vi "运维调试.vi"() -> ()   [LabVIEW 2016, in "重金属.lvlib"]
uses:
  <vilib>/Plasmionique/MB Master/MB_Master/MB_Master.lvclass
  <vilib>/Utility/miscctls.llb/LVPointTypeDef.ctl
  <userlib>/_OpenG.lib/array/array.llb/Remove Duplicates from 1D Array (String)__ogtk.vi
  <vilib>/Utility/config.llb/NI_LVConfig.lvlib
panel:
  out "MB session out":refnum<class "MB_Master.lvclass">
  out "测量结果":T1 {"汞" format="%.5f"; "锰" format="%.5f"; "镍" format="%.5f"; "锌" format="%.5f"; "铜" format="%.5f"; "镉" format="%.5f"; "铅" format="%.5f"}
  in  "参数选择配置":T2 {"通道4" items=["不启用", "铅", "镉", "铜", "锌", "镍", "锰", "汞"]; "通道3" items=["不启用", "铅", "镉", "铜", "锌", "镍", "锰", "汞"]; "通道2" items=["不启用", "铅", "镉", "铜", "锌", "镍", "锰", "汞"]; "通道1" items=["不启用", "铅", "镉", "铜", "锌", "镍", "锰", "汞"]}
  out "字符串":string
  in  "测试时间设置":dbl
  out "通讯状态":bool
  in  "设置":bool
  in  "停止":bool
  in  "启动":bool
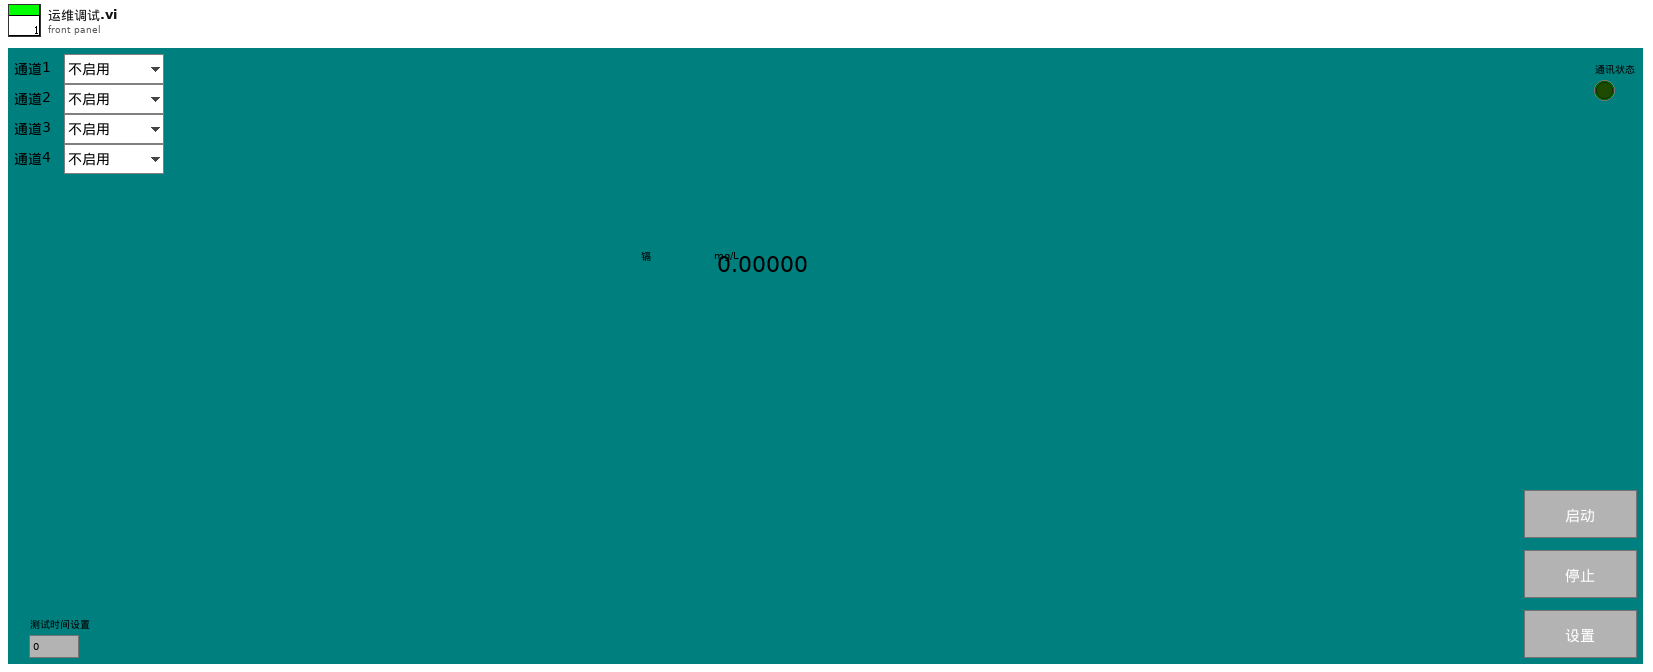
[diagram p1: front panel]
types:
  T1 = cluster{"铅":sgl, "镉":sgl, "铜":sgl, "锌":sgl, "镍":sgl, "锰":sgl, "汞":sgl}
  T2 = cluster{"通道1":u16, "通道2":u16, "通道3":u16, "通道4":u16}
  T3 = typedef "LVPointTypeDef.ctl" = cluster{"Horizontal":i16, "Vertical":i16}
  T4 = typedef "NI_LVConfig.lvlib/Config Data RefNum.ctl" = refnum<k1>
  T5 = cluster{"连接类型":enum16{"串口", "TCP"}, "串口":string, "IP":string, "PORT":string}
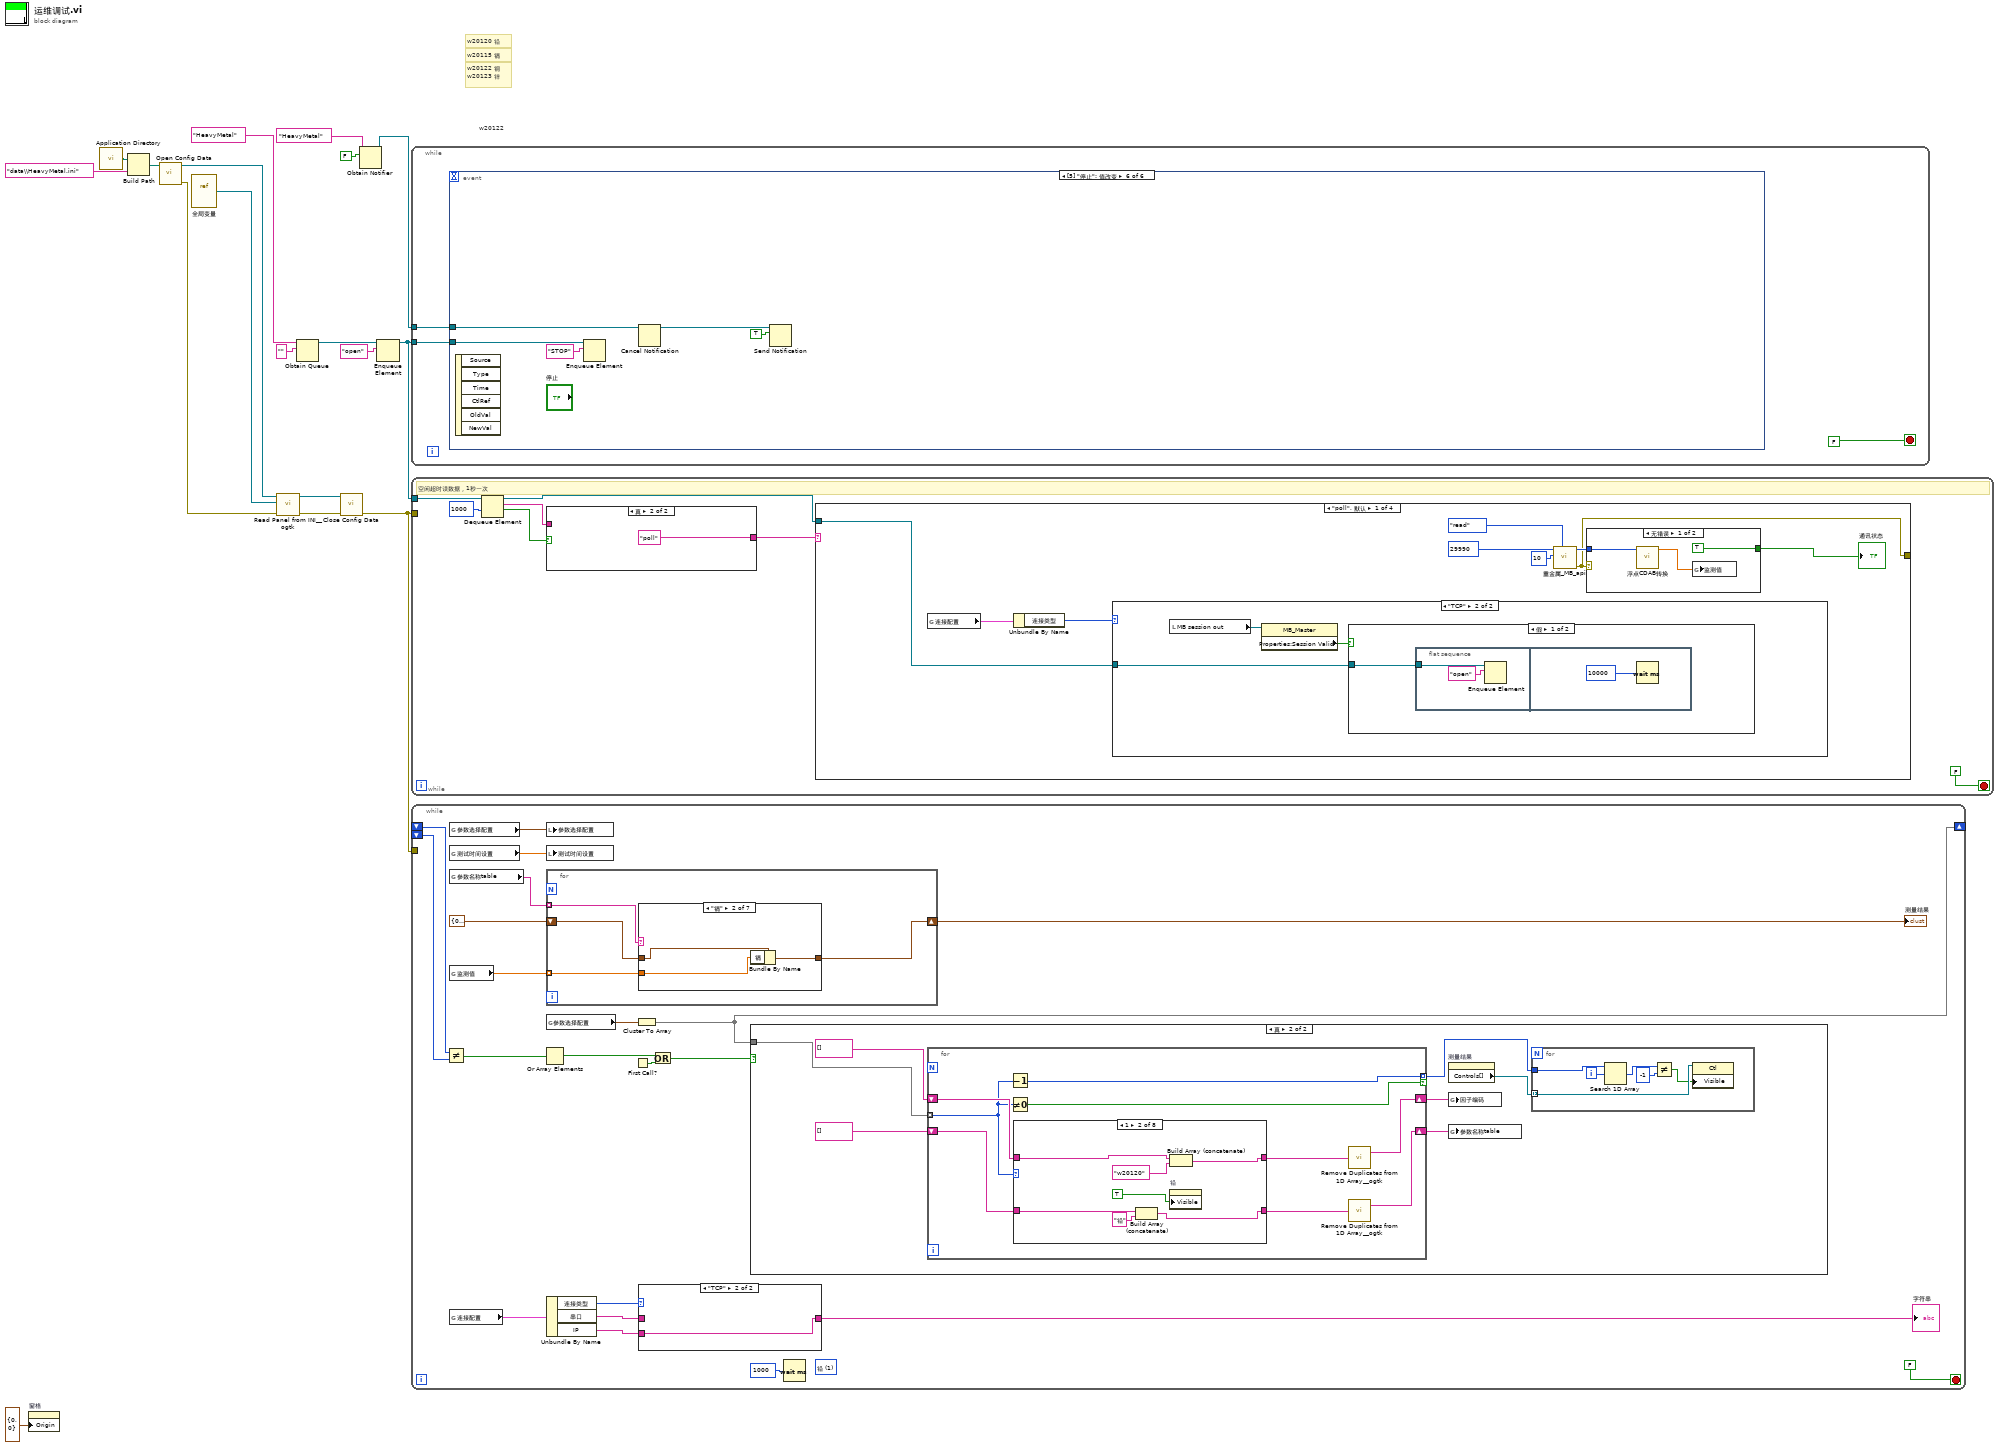
[diagram p0: block diagram]
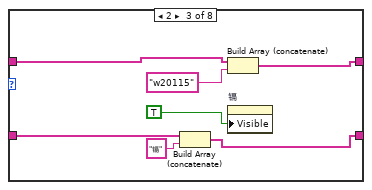
[diagram p4: hidden frame]
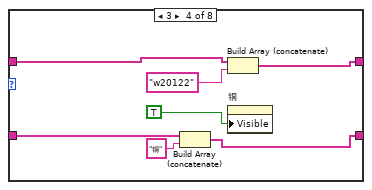
[diagram p5: hidden frame]
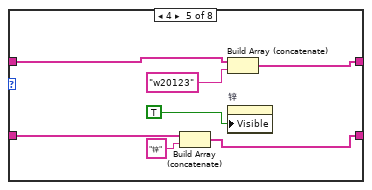
[diagram p6: hidden frame]
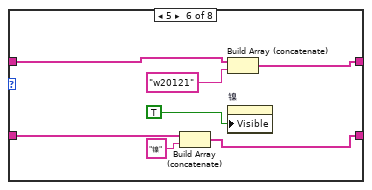
[diagram p7: hidden frame]
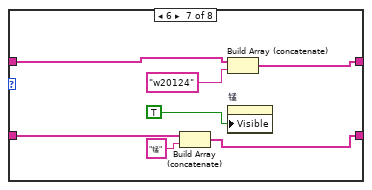
[diagram p8: hidden frame]
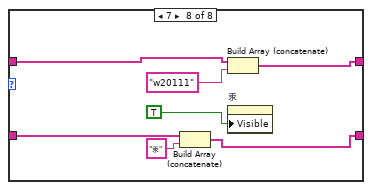
[diagram p9: hidden frame]
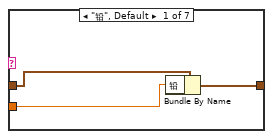
[diagram p11: hidden frame]
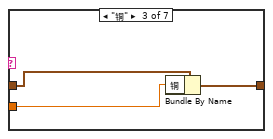
[diagram p12: hidden frame]
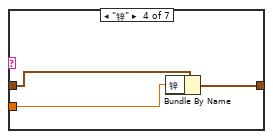
[diagram p13: hidden frame]
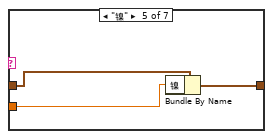
[diagram p14: hidden frame]
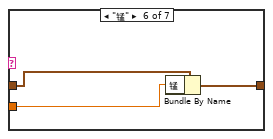
[diagram p15: hidden frame]
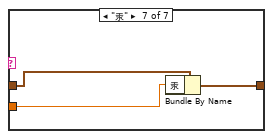
[diagram p16: hidden frame]
diagram:
  # "w20115\t镉"
  # "w20120\t铅"
  # "w20122\t铜\nw20123\t锌"
  # "w20122"
  n1 = property on="窗格" class="Pane"("Origin"=T3 {"Horizontal"=0, "Vertical"=0} ("原点")) -> ()  [unwired: 2 in, 2 out]
  n2 = call <vilib>:"Application Directory.vi"() -> ("Application Directory"=w6:path)
  n3 = Build Path(base path=w6, name or relative path="data\\HeavyMetal.ini" ("名称或相对路径")) -> (appended path=w8:path)
  n4 = call <vilib>:"Open Config Data.vi"("configuration file path"=w8) -> ("error out"=w4:errorcluster, "refnum"=w9:T4)  [unwired: 8 in, 1 out]
  n5 = vi-ref "全局变量.vi"() -> (w10:refnum<vi>)
  n6 = call <userlib>:"Read Panel from INI__ogtk.vi"("error in (no error)"=w4, "VI ref"=w10, "refnum"=w9) -> ("error out"=w5:errorcluster, "refnum out"=w11:T4)  [unwired: 7 in]
  n7 = Obtain Queue(name (unnamed)="HeavyMetal" ("名称（未命名）"), element data type="" ("元素")) -> (queue out=w15:refnum<queue>)  [unwired: 3 in, 2 out]
  n8 = call <vilib>:"Close Config Data.vi"("error in (no error)"=w5, "refnum"=w11) -> ("error out"=w1:errorcluster)  [unwired: 8 in, 1 out]
  n9 = Obtain Notifier(name (unnamed)="HeavyMetal" ("名称（未命名）"), notification data type=FALSE) -> (notifier out=w12:refnum<notifier>)  [unwired: 2 in, 2 out]
  n10 = Enqueue Element(queue=w15, element="open" ("元素")) -> (queue out=w3:refnum<queue>)  [unwired: 2 in, 2 out]
  n11 = while {
    tunnel: w3 -> [w20]
    tunnel: w12 -> [w19]
    stop <- FALSE stop-if-true
    n12 = event shown="[5] \"停止\": 值改变" {
      selector: _ -> [_ _ _ _ _ _]
      dyn-events: _ -> [_ _ _ _ _ _]
      timeout: _ -> [_ _ _ _ _ _]
      tunnel: w20 -> [_ _ _ w42 w64 w69]
      tunnel: w19 -> [_ _ _ _ _ w68]
      event Timeout {
        n13 = event-data() -> ()  [unwired: 1 in, 3 out]
      }
      event "测试时间设置": Mouse Down {
        n14 = event-data() -> ("CtlRef"=w25:refnum<vi>)  [unwired: 1 in, 7 out]
        n15 = property class="DigNum (严格)"(reference=w25) -> (reference out=w24:refnum<vi>, "Value"=w22:dbl)  [unwired: 1 in, 1 out]
        n16 = call "数字键盘.vi"("OldNumber"=w22) -> ("NewNumber"=w23:sgl)
        n17 = property class="DigNum (严格)"(reference=w24, "Val(Sgnl)"=w23) -> ()  [unwired: 1 in, 2 out]
      }
      event "测试时间设置", "参数选择配置": Value Change {
        n18 = event-data() -> ()  [unwired: 1 in, 6 out]
        n19 = flat-sequence {
          frame #0 {
            n20 = global write "全局变量.vi" "测试时间设置"("测试时间设置") -> ()
            n21 = global write "全局变量.vi" "参数选择配置"("参数选择配置") -> ()
          }
          frame #1 {
            n22 = call <vilib>:"Application Directory.vi"() -> ("Application Directory"=w41:path)
            n23 = Build Path(base path=w41, name or relative path="data\\HeavyMetal.ini" ("名称或相对路径")) -> (appended path=w39:path)
            n24 = call <vilib>:"Open Config Data.vi"("configuration file path"=w39) -> ("error out"=w35:errorcluster, "refnum"=w38:T4)  [unwired: 8 in, 1 out]
            n25 = vi-ref "全局变量.vi"() -> (w37:refnum<vi>)
            n26 = call <userlib>:"Write Panel to INI__ogtk.vi"("error in (no error)"=w35, "VI ref"=w37, "refnum"=w38) -> ("error out"=w34:errorcluster, "refnum out"=w36:T4)  [unwired: 7 in]
            n27 = call <vilib>:"Close Config Data.vi"("error in (no error)"=w34, "refnum"=w36) -> ("error out"=w29:errorcluster, "file path"=w28:path)  [unwired: 8 in]
            n28 = Open/Create/Replace File(file path (use dialog)=w28, error in=w29) -> (refnum out=w32:refnum<file>, error out=w33:errorcluster)  [unwired: 4 in, 1 out]
            n29 = Flush File(refnum=w32, error in=w33) -> (refnum out=w31:refnum<file>, error out=w30:errorcluster)
            n30 = Close File(refnum=w31, error in=w30) -> ()  [unwired: 2 out]
          }
        }
      }
      event "设置": Value Change {
        n31 = event-data() -> ()  [unwired: 1 in, 6 out]
        n32 = call "设置窗口.vi"() -> ("连接配置"=w44:T5, "确定输出"=w43:bool)  [unwired: 10 in]
        n33 = case shown="真" w43 {
          tunnel: w44 -> [_ w46]
          tunnel: w42 -> [_ w45]
          frame False {
          }
          frame True {
            n34 = flat-sequence {
              tunnel: w46 -> [w49]
              tunnel: w45 -> [w48]
              frame #0 {
                n35 = global write "全局变量.vi" "连接配置"(w49) -> ()
                n36 = Enqueue Element(queue=w48, element="open" ("元素")) -> ()  [unwired: 2 in, 3 out]
              }
              frame #1 {
                n37 = call <vilib>:"Application Directory.vi"() -> ("Application Directory"=w63:path)
                n38 = Build Path(base path=w63, name or relative path="data\\HeavyMetal.ini" ("名称或相对路径")) -> (appended path=w61:path)
                n39 = call <vilib>:"Open Config Data.vi"("configuration file path"=w61) -> ("error out"=w57:errorcluster, "refnum"=w60:T4)  [unwired: 8 in, 1 out]
                n40 = vi-ref "全局变量.vi"() -> (w59:refnum<vi>)
                n41 = call <userlib>:"Write Panel to INI__ogtk.vi"("error in (no error)"=w57, "VI ref"=w59, "refnum"=w60) -> ("error out"=w56:errorcluster, "refnum out"=w58:T4)  [unwired: 7 in]
                n42 = call <vilib>:"Close Config Data.vi"("error in (no error)"=w56, "refnum"=w58) -> ("error out"=w51:errorcluster, "file path"=w50:path)  [unwired: 8 in]
                n43 = Open/Create/Replace File(file path (use dialog)=w50, error in=w51) -> (refnum out=w54:refnum<file>, error out=w55:errorcluster)  [unwired: 4 in, 1 out]
                n44 = Flush File(refnum=w54, error in=w55) -> (refnum out=w53:refnum<file>, error out=w52:errorcluster)
                n45 = Close File(refnum=w53, error in=w52) -> ()  [unwired: 2 out]
              }
            }
          }
        }
      }
      event "启动": Value Change {
        n46 = event-data() -> ()  [unwired: 1 in, 6 out]
        n47 = Enqueue Element(queue=w64, element="start" ("元素")) -> ()  [unwired: 2 in, 3 out]
      }
      event "停止": Value Change {
        n48 = event-data() -> ()  [unwired: 1 in, 6 out]
        n49 = Enqueue Element(queue=w69, element="STOP" ("元素")) -> ()  [unwired: 2 in, 3 out]
        n50 = Cancel Notification(0:w68) -> (8:w66:refnum<notifier>)  [unwired: 1 in, 2 out]
        n51 = Send Notification(notification=TRUE, notifier=w66) -> ()  [unwired: 1 in, 2 out]
      }
    }
  }
  n52 = while {
    tunnel: w3 -> [w77]
    tunnel: w1 -> [_]
    stop <- FALSE stop-if-true
    # "空闲超时读数据，1秒一次"
    n53 = Dequeue Element(queue=w77, timeout in ms (-1)=1000 ("超时毫秒(-1)")) -> (queue out=w71:refnum<queue>, element=w74:string, timed out?=w75:bool)  [unwired: 1 in, 1 out]
    n54 = case shown="真" w75 {
      tunnel: w74 -> [w78 _]
      tunnel: [w78 "poll" ("元素")] -> w73
      frame False {
      }
      frame True {
      }
    }
    n55 = case shown="\"poll\", 默认" w73 {
      tunnel: [w84 w100 w105 w109] -> _
      tunnel: w71 -> [w80 _ _ _]
      frame "poll", Default {
        n56 = global read "全局变量.vi" "连接配置"() -> (w82:T5)
        n57 = Unbundle By Name(w82) -> ("连接类型"=w81:enum16{"串口", "TCP"})
        n58 = case shown="\"TCP\"" w81 {
          tunnel: w80 -> [_ w89]
          frame "串口", Default {
          }
          frame "TCP" {
            n59 = local read "MB session out"() -> (w91:refnum<class "MB_Master.lvclass">)
            n60 = property class="MB_Master"(reference=w91) -> ("Properties:Session Valid"=w90:bool)  [unwired: 1 in, 2 out]
            n61 = case shown="假" w90 {
              tunnel: w89 -> [w92 _]
              frame False {
                n62 = flat-sequence {
                  tunnel: w92 -> [w94]
                  frame #0 {
                    n63 = Enqueue Element(queue=w94, element="open" ("元素")) -> ()  [unwired: 2 in, 3 out]
                  }
                  frame #1 {
                    n64 = Wait (ms)(milliseconds to wait=u32 10000 ("等待时间（毫秒）")) -> ()  [unwired: 1 out]
                  }
                }
              }
              frame True {
              }
            }
          }
        }
        n65 = call "重金属_MB_api.vi"("STEP"=enum16{"open", "read", "write", "close"}."read", "quantity"=u16 10, "starting address"=u16 29990) -> ("error out"=w84:errorcluster, "Registers"=w85:u16[])  [unwired: 5 in, 2 out]
        n66 = case shown="无错误" w84 {
          tunnel: w85 -> [w98 _]
          tunnel: [TRUE ("通讯状态") _] -> w83
          frame No Error {
            n67 = call "浮点CDAB转换.vi"("数组"=w98) -> ("数组 2"=w96:sgl[])  [unwired: 10 in]
            n68 = global write "全局变量.vi" "监测值"(w96) -> ()
          }
          frame Error {
          }
        }
        "通讯状态" <- w83
      }
      frame "open" {
        n69 = global read "全局变量.vi" "连接配置"() -> (w102:T5)
        n70 = call "重金属_MB_api.vi"("连接配置"=w102, "STEP"=enum16{"open", "read", "write", "close"}."open") -> ("error out"=w100:errorcluster, "MB session out"=→"MB session out":refnum<class "MB_Master.lvclass">)  [unwired: 6 in, 2 out]
      }
      frame "start" {
        n71 = call "重金属_MB_api.vi"("STEP"=enum16{"open", "read", "write", "close"}."write", "values"=u16 1, "starting address"=u16 29980) -> ("error out"=w105:errorcluster)  [unwired: 5 in, 3 out]
      }
      frame "stop" {
        n72 = global read "全局变量.vi" "连接配置"() -> (w111:T5)
        n73 = call "重金属_MB_api.vi"("连接配置"=w111, "STEP"=enum16{"open", "read", "write", "close"}."write", "values"=u16 1, "starting address"=u16 29989) -> ("error out"=w109:errorcluster)  [unwired: 4 in, 3 out]
      }
    }
  }
  n74 = while {
    tunnel: w1 -> [_]
    shift-right: [w118] -> _
    shift-left: _ -> [w116]
    shift-left: _ -> [w117]
    stop <- FALSE stop-if-true
    (unwired) u16 1 items=["不启用", "铅", "镉", "铜", "锌", "镍", "锰", "汞"] ("通道1")
    n75 = Not Equal?(x=w116, y=w117) -> (x != y?=w115:bool[])
    n76 = global read "全局变量.vi" "参数选择配置"() -> (w129:T2)
    n77 = global read "全局变量.vi" "测试时间设置"() -> (w130:dbl)
    n78 = global read "全局变量.vi" "参数名称table"() -> (w127:string[])
    n79 = global read "全局变量.vi" "监测值"() -> (w125:dbl[])
    n80 = global read "全局变量.vi" "连接配置"() -> (w119:T5)
    n81 = Or Array Elements(Boolean array=w115) -> (logical OR=w114:bool)
    n82 = local write "参数选择配置"(w129) -> ()
    n83 = local write "测试时间设置"(w130) -> ()
    n84 = for {
      tunnel: w127 -> [w211] mode=indexing
      shift-right: [w209] -> w126
      shift-left: T1 {"铅"=0.0, "镉"=0.0, "铜"=0.0, "锌"=0.0, "镍"=0.0, "锰"=0.0, "汞"=0.0} ("测量结果") -> [w210]
      tunnel: w125 -> [w208] mode=indexing
      n85 = case shown="\"镉\"" w211 {
        tunnel: w210 -> [w214 w217 w219 w222 w225 w228 w232]
        tunnel: [w213 w215 w218 w221 w224 w227 w230] -> w209
        tunnel: w208 -> [w212 w216 w220 w223 w226 w229 w231]
        frame "铅", Default {
          n86 = Bundle By Name(cluster=w214, "铅"=w212) -> (w213:T1)
        }
        frame "镉" {
          n87 = Bundle By Name(cluster=w217, "镉"=w216) -> (w215:T1)
        }
        frame "铜" {
          n88 = Bundle By Name(cluster=w219, "铜"=w220) -> (w218:T1)
        }
        frame "锌" {
          n89 = Bundle By Name(cluster=w222, "锌"=w223) -> (w221:T1)
        }
        frame "镍" {
          n90 = Bundle By Name(cluster=w225, "镍"=w226) -> (w224:T1)
        }
        frame "锰" {
          n91 = Bundle By Name(cluster=w228, "锰"=w229) -> (w227:T1)
        }
        frame "汞" {
          n92 = Bundle By Name(cluster=w232, "汞"=w231) -> (w230:T1)
        }
      }
    }
    "测量结果" <- w126
    n93 = global read "全局变量.vi" "参数选择配置"() -> (w128:T2)
    n94 = Unbundle By Name(w119) -> ("连接类型"=w120:enum16{"串口", "TCP"}, "串口"=w123:string, "IP"=w122:string)
    n95 = First Call?() -> (First Call?: T/F=w112:bool)
    n96 = Cluster To Array(cluster=w128) -> (array=w118:u16[])
    n97 = case shown="\"TCP\"" w120 {
      tunnel: [w206 w207] -> w121
      tunnel: w122 -> [_ w207]
      tunnel: w123 -> [w206 _]
      frame "串口", Default {
      }
      frame "TCP" {
      }
    }
    "字符串" <- w121
    n98 = Or(x=w114, y=w112) -> (x .or. y?=w113:bool)
    n99 = case shown="真" w113 {
      tunnel: w118 -> [_ w135]
      frame False {
      }
      frame True {
        n100 = for {
          tunnel: w135 -> [w147] mode=indexing
          shift-right: [w151] -> w138
          shift-left: string[] [] -> [w154]
          shift-right: [w149] -> w136
          shift-left: string[] [] -> [w153]
          tunnel: [w148] -> w133 mode=indexing if=w146
          n101 = Decrement(x=w147) -> (x-1=w148:u16)
          n102 = Not Equal To 0?(x=w147) -> (x != 0?=w146:bool)
          n103 = case shown="1" w147 {
            tunnel: [w156 w160 w167 w174 w181 w188 w195 w202] -> w152
            tunnel: w154 -> [w156 w162 w169 w176 w183 w190 w197 w204]
            tunnel: w153 -> [w155 w159 w165 w172 w179 w186 w193 w200]
            tunnel: [w155 w158 w164 w171 w178 w185 w192 w199] -> w150
            frame 0, Default {
            }
            frame 1 {
              n104 = Build Array (concatenate)(w162, "铅") -> (w160:string[])
              n105 = Build Array (concatenate)(w159, "w20120") -> (w158:string[])
              n106 = property on="铅" class="DigNum (严格)"("Visible"=TRUE ("可见")) -> ()  [unwired: 2 in, 2 out]
            }
            frame 2 {
              n107 = Build Array (concatenate)(w169, "镉") -> (w167:string[])
              n108 = Build Array (concatenate)(w165, "w20115") -> (w164:string[])
              n109 = property on="镉" class="DigNum (严格)"("Visible"=TRUE ("可见")) -> ()  [unwired: 2 in, 2 out]
            }
            frame 3 {
              n110 = Build Array (concatenate)(w176, "铜") -> (w174:string[])
              n111 = Build Array (concatenate)(w172, "w20122") -> (w171:string[])
              n112 = property on="铜" class="DigNum (严格)"("Visible"=TRUE ("可见")) -> ()  [unwired: 2 in, 2 out]
            }
            frame 4 {
              n113 = Build Array (concatenate)(w183, "锌") -> (w181:string[])
              n114 = Build Array (concatenate)(w179, "w20123") -> (w178:string[])
              n115 = property on="锌" class="DigNum (严格)"("Visible"=TRUE ("可见")) -> ()  [unwired: 2 in, 2 out]
            }
            frame 5 {
              n116 = Build Array (concatenate)(w190, "镍") -> (w188:string[])
              n117 = Build Array (concatenate)(w186, "w20121") -> (w185:string[])
              n118 = property on="镍" class="DigNum (严格)"("Visible"=TRUE ("可见")) -> ()  [unwired: 2 in, 2 out]
            }
            frame 6 {
              n119 = Build Array (concatenate)(w197, "锰") -> (w195:string[])
              n120 = Build Array (concatenate)(w193, "w20124") -> (w192:string[])
              n121 = property on="锰" class="DigNum (严格)"("Visible"=TRUE ("可见")) -> ()  [unwired: 2 in, 2 out]
            }
            frame 7 {
              n122 = Build Array (concatenate)(w204, "汞") -> (w202:string[])
              n123 = Build Array (concatenate)(w200, "w20111") -> (w199:string[])
              n124 = property on="汞" class="DigNum (严格)"("Visible"=TRUE ("可见")) -> ()  [unwired: 2 in, 2 out]
            }
          }
          n125 = call-poly <userlib>:"Remove Duplicates from 1D Array__ogtk.vi"("Input Array"=w150) -> ("Output Array"=w149:string[])  [unwired: 1 out]
          n126 = call-poly <userlib>:"Remove Duplicates from 1D Array__ogtk.vi"("Input Array"=w152) -> ("Output Array"=w151:string[])  [unwired: 1 out]
        }
        n127 = property on="测量结果" class="Clust (严格)"() -> ("Controls[]"=w134:refnum<vi>[])  [unwired: 2 in, 2 out]
        n128 = global write "全局变量.vi" "因子编码"(w136) -> ()
        n129 = global write "全局变量.vi" "参数名称table"(w138) -> ()
        n130 = for {
          tunnel: w134 -> [w145] mode=indexing
          tunnel: w133 -> [w144]
          i -> [w143]
          n131 = Search 1D Array(1D array=w144, element=w143) -> (index of element=w142:i32)  [unwired: 1 in]
          n132 = Not Equal?(x=w142, y=-1) -> (x != y?=w140:bool)
          n133 = property class="Ctl"(reference=w145, "Visible"=w140) -> ()  [unwired: 1 in, 2 out]
        }
      }
    }
    n134 = Wait (ms)(milliseconds to wait=u32 1000 ("等待时间（毫秒）")) -> ()  [unwired: 1 out]
  }
